vi "Determine Warnings.vi"() -> ()   [LabVIEW 2014]
panel:
  out "Warning?":bool
  out "Warning Text":string
  in  "Min Temp":dbl
  in  "Max Temp":dbl
  in  "Current Temp":dbl
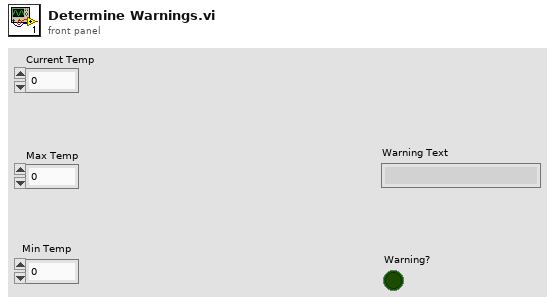
[diagram p1: front panel]
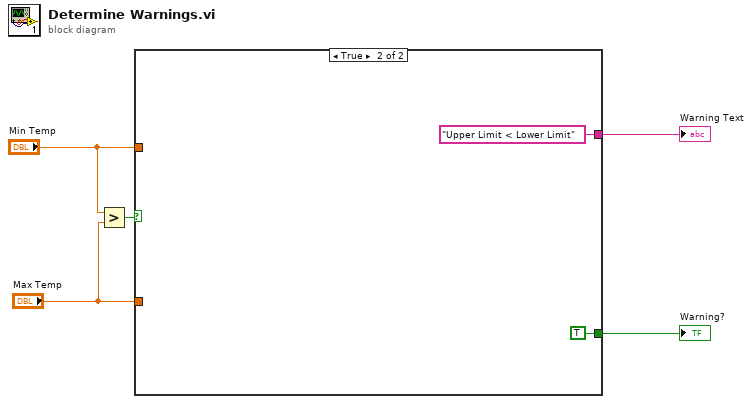
[diagram p0: block diagram]
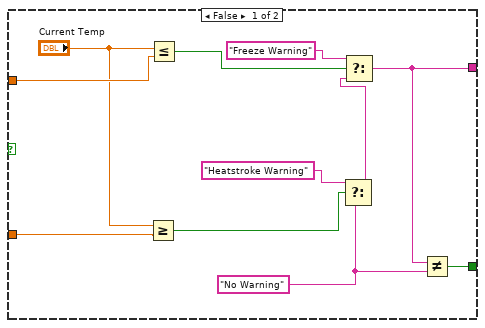
[diagram p2: hidden frame]
diagram:
  n1 = Greater?(x="Min Temp", y="Max Temp") -> (0:w3:bool)
  n2 = case shown="True" w3 {
    tunnel: [w13 "Upper Limit < Lower Limit"] -> w5
    tunnel: [w12 TRUE] -> w4
    tunnel: "Max Temp" -> [w8 _]
    tunnel: "Min Temp" -> [w7 _]
    frame False {
      w14 = "No Warning"
      n3 = Greater Or Equal?(x="Current Temp", y=w8) -> (x >= y?=w10:bool)
      n4 = Less Or Equal?(x="Current Temp", y=w7) -> (x <= y?=w9:bool)
      n5 = Select(t="Heatstroke Warning", s=w10, f=w14) -> (s? t:f=w11:string)
      n6 = Select(t="Freeze Warning", s=w9, f=w11) -> (s? t:f=w13:string)
      n7 = Not Equal?(x=w13, y=w14) -> (x != y?=w12:bool)
    }
    frame True {
    }
  }
  "Warning Text" <- w5
  "Warning?" <- w4
